vi "TcA01-002_ObjectCreationAndDestructionOfSubclass.vi"(1 "Input buffer":T3="1", 3 "Invocation info":T2, 5 "error in (no error)":errorcluster, 6 "Add log to result?":bool) -> (16 "Test Data":T1 {"Numeric Measurement" format="%.2f"}, 19 "error out":errorcluster)   [LabVIEW 2020]
doc: "Test case template."
uses:
  Shared/Support_InputBuffer.ctl
  Shared/Support_InvocationInfo.ctl
  Shared/Support_TestData.ctl
  TestClasses/G#SubClass1_class/G#SubClass1.lvclass
  <vilib>/addons/_AddQ/G#Object/G#Object.lvclass
panel:
  in  "Test name":string="TcA01-002 Object creation and destruction of sub class"
  out "Test result":bool
  out "Result":string
  # "Verify that multiple objects of a sub class can\nbe created and destructed multiple times."
  # "Sub test case"
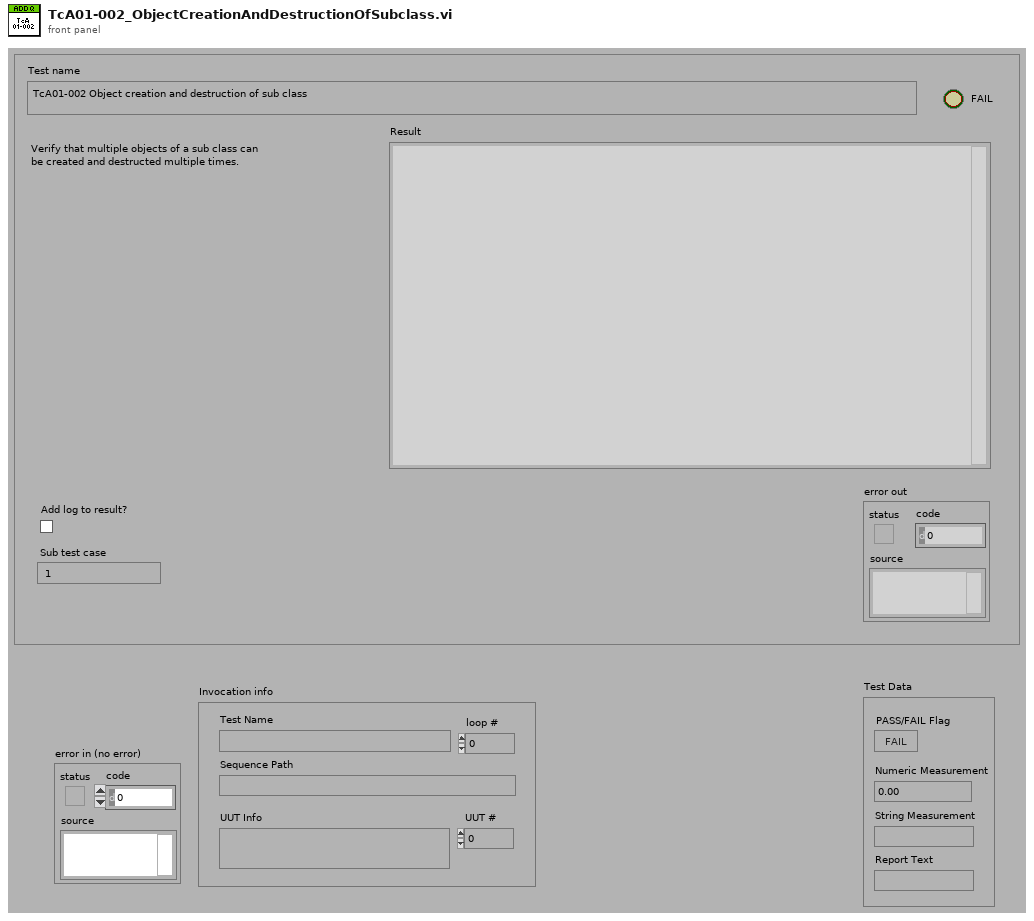
[diagram p1: front panel]
types:
  T1 = typedef "Support_TestData.ctl" = cluster{"PASS/FAIL Flag":bool, "Numeric Measurement":dbl, "String Measurement":string, "Report Text":string}
  T2 = typedef "Support_InvocationInfo.ctl" = cluster{"UUT #":i32, "loop #":i32, "UUT Info":string, "Test Name":string, "Sequence Path":path}
  T3 = typedef "Support_InputBuffer.ctl" = string
  T4 = typedef "Support_ResultType.ctl" = cluster{"Pass":bool, "Comment":string, "MeasurementValue":dbl}
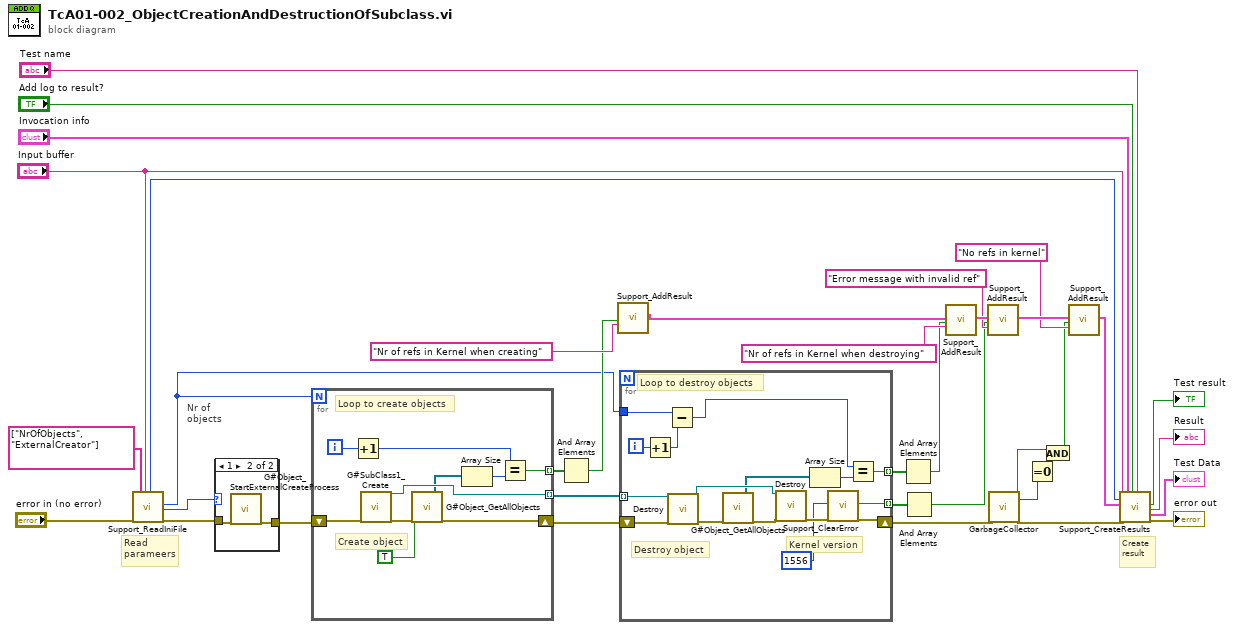
[diagram p0: block diagram]
diagram:
  # "Read\nparameers"
  # "Create\nresult"
  # "Nr of\nobjects"
  n1 = call "Support_ReadIniFile.vi"("error in (no error)"="error in (no error)", "Parameter names"=string[] ["NrOfObjects", "ExternalCreator"], "Sub test case"="Input buffer") -> ("Timer start"=w20:u32, "Parameter1 as I32"=w3:i32, "Parameter2 as I32"=w2:i32, "error out"=w5:errorcluster)  [unwired: 9 in, 4 out]
  n2 = case shown="1" w2 {
    tunnel: w5 -> [w38 w40]
    tunnel: [w38 w39] -> w4
    frame 0, Default {
    }
    frame 1 {
      n3 = call <vilib>:"G#Object_StartExternalCreateProcess.vi"("error in (no error)"=w40) -> ("error out"=w39:errorcluster)  [unwired: 18 in]
    }
  }
  n4 = for {
    N: w3 -> [_]
    shift-right: [w41] -> w27
    shift-left: w4 -> [w50]
    tunnel: [w44] -> w26 mode=indexing
    tunnel: [w46] -> w30 mode=indexing
    i -> [w49]
    # "Create object"
    # "Loop to create objects"
    n5 = Increment(x=w49) -> (x+1=w47:i32)
    n6 = call "G#SubClass1_Create.vi"("error in (no error)"=w50) -> ("reference out"=w44:refnum<class "G#SubClass1.lvclass">, "error out"=w45:errorcluster)  [unwired: 16 in, 1 out]
    n7 = call <vilib>:"G#Object_GetAllObjects.vi"("only refs (F)"=TRUE ("only refs"), "error in (no error)"=w45) -> ("all refs"=w43:refnum<class "G#Object.lvclass">[], "error out"=w41:errorcluster)  [unwired: 14 in, 2 out]
    n8 = Array Size(array=w43) -> (size(s)=w48:i32)
    n9 = Equal?(x=w47, y=w48) -> (x = y?=w46:bool)
  }
  n10 = And Array Elements(Boolean array=w30) -> (logical AND=w28:bool)
  n11 = call "Support_AddResult.vi"("Pass"=w28, "Comment"="Nr of refs in Kernel when creating") -> ("Results out"=w15:T4[])  [unwired: 17 in]
  n12 = for {
    shift-right: [w56] -> w14
    shift-left: w27 -> [w64]
    tunnel: [w65] -> w25 mode=indexing
    tunnel: w26 -> [w60] mode=indexing
    tunnel: w3 -> [w63]
    tunnel: [w55] -> w19 mode=indexing
    i -> [w66]
    # "Destroy object"
    # "Loop to destroy objects"
    # "Kernel version"
    n13 = Increment(x=w66) -> (x+1=w62:i32)
    n14 = Subtract(x=w63, y=w62) -> (x-y=w61:i32)
    n15 = call-dynamic "Destroy.vi"("reference in"=w60, "error in (no error)"=w64) -> ("reference out"=w54:refnum<class "G#SubClass1.lvclass">, "error out"=w51:errorcluster)  [unwired: 16 in]
    n16 = call <vilib>:"G#Object_GetAllObjects.vi"("error in (no error)"=w51) -> ("all refs"=w52:refnum<class "G#Object.lvclass">[], "error out"=w53:errorcluster)  [unwired: 15 in, 2 out]
    n17 = call-dynamic "Destroy.vi"("reference in"=w54, "error in (no error)"=w53) -> ("error out"=w58:errorcluster)  [unwired: 16 in, 1 out]
    n18 = Array Size(array=w52) -> (size(s)=w59:i32)
    n19 = call "Support_ClearError.vi"("code"=1556, "error in (no error)"=w58) -> ("Cleared?"=w55:bool, "error out"=w56:errorcluster)  [unwired: 16 in]
    n20 = Equal?(x=w61, y=w59) -> (x = y?=w65:bool)
  }
  n21 = And Array Elements(Boolean array=w25) -> (logical AND=w23:bool)
  n22 = And Array Elements(Boolean array=w19) -> (logical AND=w16:bool)
  n23 = call "Support_AddResult.vi"("Results in"=w15, "Pass"=w23, "Comment"="Nr of refs in Kernel when destroying") -> ("Results out"=w18:T4[])  [unwired: 16 in]
  n24 = call "Support_AddResult.vi"("Results in"=w18, "Pass"=w16, "Comment"="Error message with invalid ref") -> ("Results out"=w12:T4[])  [unwired: 16 in]
  n25 = call <vilib>:"GarbageCollector.vi"("error in (no error)"=w14) -> ("OK"=w9:bool, "# of objects killed"=w7:i32, "error out"=w13:errorcluster)  [unwired: 16 in]
  n26 = Equal To 0?(x=w7) -> (x = 0?=w8:bool)
  n27 = And(x=w9, y=w8) -> (x .and. y?=w6:bool)
  n28 = call "Support_AddResult.vi"("Results in"=w12, "Pass"=w6, "Comment"="No refs in kernel") -> ("Results out"=w11:T4[])  [unwired: 16 in]
  n29 = call "Support_CreateResults.vi"("Sub test case"="Input buffer", "Timer start"=w20, "Results"=w11, "error in (no error)"=w13, "Invocation info"="Invocation info", "Add log to result?"="Add log to result?", "Test name"="Test name") -> ("Pass/fail flag"=→"Test result":bool, "Result"=→"Result":string, "Test Data"=→"Test Data":T1, "error out"=→"error out":errorcluster)  [unwired: 9 in]
